vi "Selection.Convert.Get.vi"(8 "error in (no error)":errorcluster, 11 "ListBox in":refnum<vi>) -> (0 "error out":errorcluster, 2 "Analysis Options":T1={"Pull In Time"=TRUE, "Pull In Max Current"=TRUE, "Pull In Max Voltage"=TRUE, "Pull In Min Voltage"=TRUE, "Pull In Avg Voltage"=TRUE, "Hold In Time"=TRUE, "Hold In Max Current"=TRUE, "Hold In Min Current"=TRUE, "Hold In Avg Current"=TRUE, "Hold In Max Voltage"=TRUE, "Hold In Min Voltage"=TRUE, "Hold In Avg Max Voltage"=TRUE, "Hold In Avg Min Voltage"=TRUE, "Off Time"=TRUE, "Off Stage Max Current"=TRUE, "Off Stage Min Current"=TRUE, "Off Stage Avg Current"=TRUE, "Off Stage Max Voltage"=TRUE, "Off Stage Min Voltage"=TRUE, "Off Stage Avg Voltage"=TRUE, "Total Voltage Pulses"=TRUE, "Total Stage Time"=TRUE})   [LabVIEW 2015, in "Fuel Injector Analysis Addon System Explorer.lvlib"]
uses:
  Fuel Injector Analysis Addon System Explorer.lvlib
  Shared/Types/Analysis.Channels.Select.ctl
  Shared/Fuel Injector Analysis Addon Shared.lvlib
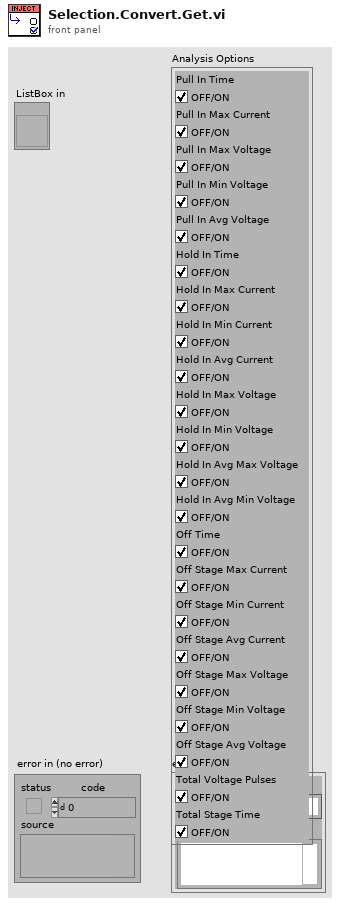
[diagram p1: front panel]
types:
  T1 = typedef "Fuel Injector Analysis Addon Shared.lvlib/Analysis.Channels.Select.ctl" = cluster{"Pull In Time":bool, "Pull In Max Current":bool, "Pull In Max Voltage":bool, "Pull In Min Voltage":bool, "Pull In Avg Voltage":bool, "Hold In Time":bool, "Hold In Max Current":bool, "Hold In Min Current":bool, "Hold In Avg Current":bool, "Hold In Max Voltage":bool, "Hold In Min Voltage":bool, "Hold In Avg Max Voltage":bool, "Hold In Avg Min Voltage":bool, "Off Time":bool, "Off Stage Max Current":bool, "Off Stage Min Current":bool, "Off Stage Avg Current":bool, "Off Stage Max Voltage":bool, "Off Stage Min Voltage":bool, "Off Stage Avg Voltage":bool, "Total Voltage Pulses":bool, "Total Stage Time":bool}
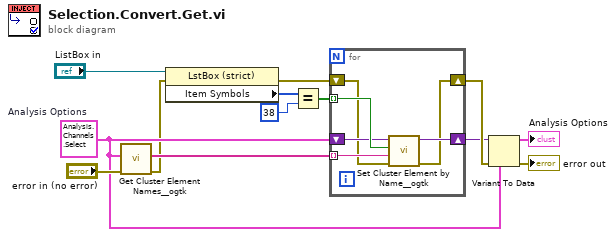
[diagram p0: block diagram]
diagram:
  w10 = T1 {"Pull In Time"=TRUE, "Pull In Max Current"=TRUE, "Pull In Max Voltage"=TRUE, "Pull In Min Voltage"=TRUE, "Pull In Avg Voltage"=TRUE, "Hold In Time"=TRUE, "Hold In Max Current"=TRUE, "Hold In Min Current"=TRUE, "Hold In Avg Current"=TRUE, "Hold In Max Voltage"=TRUE, "Hold In Min Voltage"=TRUE, "Hold In Avg Max Voltage"=TRUE, "Hold In Avg Min Voltage"=TRUE, "Off Time"=TRUE, "Off Stage Max Current"=TRUE, "Off Stage Min Current"=TRUE, "Off Stage Avg Current"=TRUE, "Off Stage Max Voltage"=TRUE, "Off Stage Min Voltage"=TRUE, "Off Stage Avg Voltage"=TRUE, "Total Voltage Pulses"=TRUE, "Total Stage Time"=TRUE}  # Analysis Options
  n1 = call <userlib>:"Get Cluster Element Names__ogtk.vi"("error in (no error)"="error in (no error)", "Cluster"=w10) -> ("error out"=w4:errorcluster, "Element Names"=w5:string[])  [unwired: 8 in]
  n2 = property class="LstBox (strict)"(reference="ListBox in", error in=w4) -> (error out=w7:errorcluster, "Item Symbols"=w2:i32[])  [unwired: 1 out]
  n3 = Equal?(x=w2, y=38) -> (x = y?=w6:bool[])
  n4 = for {
    tunnel: w5 -> [w19] mode=indexing
    tunnel: w6 -> [w18] mode=indexing
    shift-right: [w16] -> w8
    shift-left: w10 -> [w17]
    shift-right: [w14] -> w9
    shift-left: w7 -> [w15]
    n5 = call <userlib>:"Set Cluster Element by Name__ogtk.vi"("error in (no error)"=w15, "Element Name (\"\": New Element Data Name)"=w19, "New Element Value"=w18, "Cluster"=w17) -> ("error out"=w14:errorcluster, "VCluster out"=w16:variant)  [unwired: 5 in, 1 out]
  }
  n6 = Variant To Data(error in=w9, type=w10, Variant=w8) -> (data=→"Analysis Options":T1, error out=→"error out":errorcluster)
